vi "TCPReadFlush.vi"(8 "error in (no error)":errorcluster, 11 "TCP Network Connection in":refnum<k5>) -> (0 "error out":errorcluster, 3 "TCP Network Connection out":refnum<k5>)   [LabVIEW 2013]
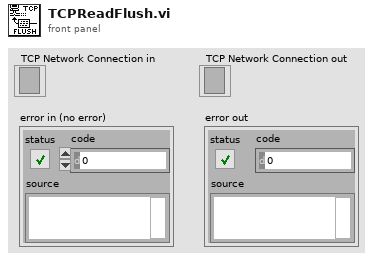
[diagram p1: front panel]
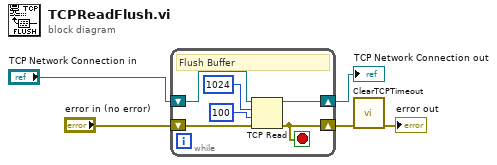
[diagram p0: block diagram]
diagram:
  n1 = while {
    shift-right: [w7] -> w5
    shift-left: "TCP Network Connection in" -> [w10]
    shift-right: [w6] -> w3
    shift-left: "error in (no error)" -> [w11]
    stop <- w6 stop-if-true
    # "Flush Buffer"
    n2 = TCP Read(connection ID=w10, bytes to read=1024, error in (no error)=w11, 9:100 ("timeout ms (25000)")) -> (connection ID out=w7:refnum<k5>, error out=w6:errorcluster)  [unwired: 1 in, 1 out]
  }
  "TCP Network Connection out" <- w5
  n3 = call "ClearTCPTimeout.vi"("error in (no error)"=w3) -> ("error out"=→"error out":errorcluster)  [unwired: 9 in, 1 out]
